vi "Strain with Nulling.vi"() -> ()   [LabVIEW 2009]
doc: "I. Description:\nThis example demonstrates how to acquire a continuous amount of data (Waveform) using the DAQ device's internal clock.\n\nII. Instructions for Running:\n1. Create an analog input voltage channel.\n2. Set the rate for the sample clock. Additionally, define the sample mode to be continuous.\n3. Call the Start VI to start the acquisition.\n4. Read the waveform data in a loop until the user hits the stop button or an error occurs.\nNote: This example reads data from one or more channels and returns an array of data. Use the Index Array function to access an individual channel of data.\n5. Call the Clear Task VI to clear the Task.\n6. Use the popup dialog box to display an error if any.\n\nIV. I/O Connections Overview:\nMake sure your signal input terminal matches the Physical Channel I/O Control. For further connection information, refer to your hardware reference manual."
uses:
  <vilib>/DAQmx/configure/timing.llb/DAQmx Timing (Sample Clock).vi
  <vilib>/DAQmx/create/channels.llb/DAQmx Create Channel (AI-Strain-Strain Gage).vi
  <vilib>/DAQmx/read.llb/DAQmx Read (Analog Wfm 1Chan NSamp).vi
  Program Files/National Instruments/LabVIEW 2009/resource/objmgr/daqmx.rc
panel:
  out "Strain Measurement":waveform(dbl)(graph)
  in  "Do Offset Nulling?":bool
  in  "Sample Rate":dbl=9.0 format="%0.2f"
  in  "strain gage information":T1={"gage factor"=2.0, "nominal gage resistance"=120.0, "poisson ratio"=0.3} {"poisson ratio" format="%0.2f"; "nominal gage resistance" format="%0.2f"; "gage factor" format="%0.2f"}
  in  "bridge information":T2={"strain configuration"=10271, "lead wire resistance"=0.0, "initial bridge voltage"=0.0, "voltage excitation source"=10200, "voltage excitation value"=2.5} {"initial bridge voltage" format="%0.2f"; "voltage excitation source" items=["Internal"=10200, "External"=10167, "None"=10230]; "voltage excitation value" format="%0.2f"; "lead wire resistance" format="%0.2f"; "strain configuration" items=["Full Bridge I"=10183, "Full Bridge II"=10184, "Full Bridge III"=10185, "Half Bridge I"=10188, "Half Bridge II"=10189, "Quarter Bridge I"=10271, "Quarter Bridge II"=10272]}
  in  "Strain Gage Channel":tag="cDAQ1Mod1/ai3" caption="Physical Channels"
  in  "minimum value (Strain)":dbl=-0.01 caption="Minimum Value" format="%0.3f"
  in  "maximum value (Strain)":dbl=0.01 caption="Maximum Value" format="%0.3f"
  in  "Samples to Read":i32=9
  in  "stop":bool
  # "Channel Parameters"
  # "Timing Parameters"
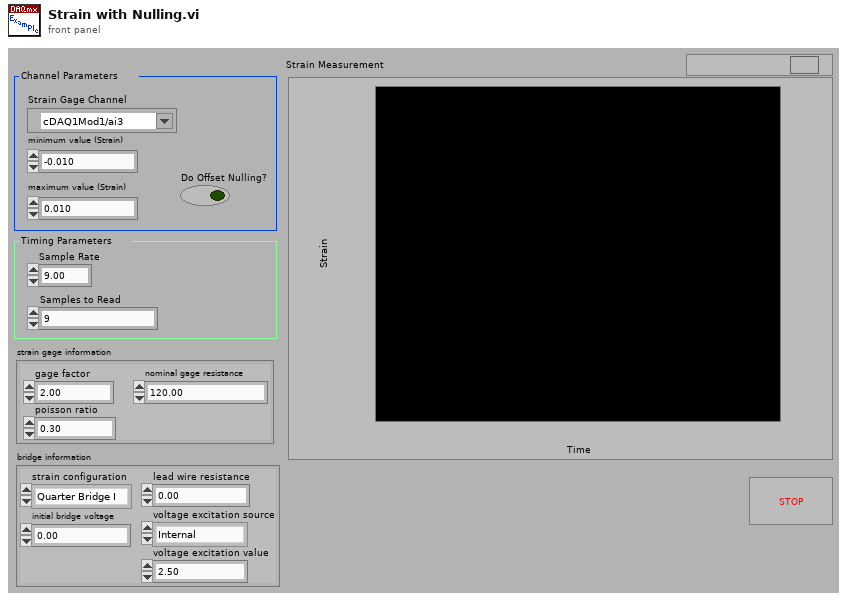
[diagram p1: front panel]
types:
  T1 = cluster{"gage factor":dbl, "nominal gage resistance":dbl, "poisson ratio":dbl}
  T2 = cluster{"strain configuration":i32, "lead wire resistance":dbl, "initial bridge voltage":dbl, "voltage excitation source":i32, "voltage excitation value":dbl}
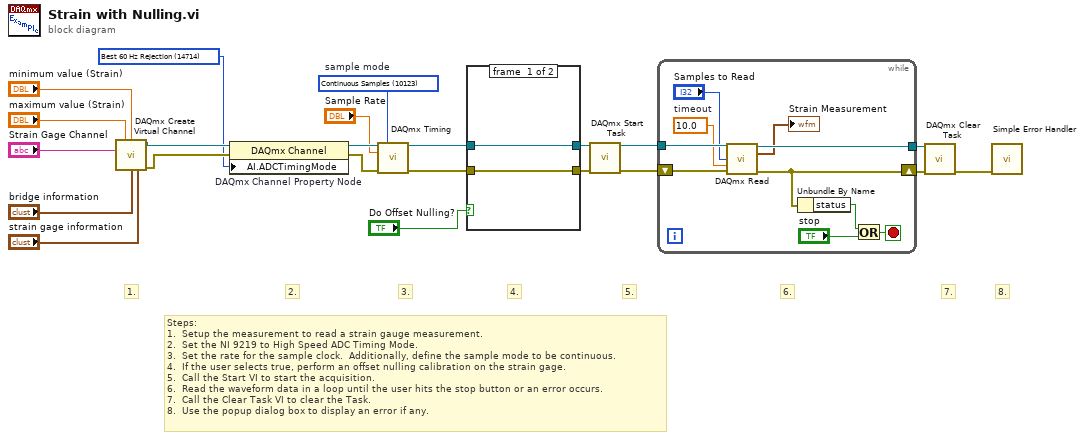
[diagram p0: block diagram]
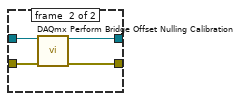
[diagram p2: hidden frame]
diagram:
  w9 = 14714 items=["High Resolution"=10195, "High Speed"=14712, "Best 50 Hz Rejection"=14713, "Best 60 Hz Rejection"=14714] ("AI.ADCTimingMode")
  w18 = 10123 items=["Finite Samples"=10178, "Continuous Samples"=10123]  # sample mode
  # "Steps: \n1.  Setup the measurement to read a strain gauge measurement.\n2.  Set the NI 9219 to High Speed ADC Timing Mode.\n3.  Set the rate for the sample clock.  Additionally, define the sample mode to be continuous.\n4.  If the user selects true, perform an offset nulling calibration on the strain gage.\n5.  Call the Start VI to start the acquisition.\n6.  Read the waveform data in a loop until the user hits the stop button or an error occurs.\n7.  Call the Clear Task VI to clear the Task.\n8.  Use the popup dialog box to display an error if any."
  # "4."
  # "6."
  # "2."
  # "8."
  # "7."
  # "5."
  # "3."
  # "1."
  n1 = call-poly <vilib>:"DAQmx Create Virtual Channel.vi"("maximum value"="maximum value (Strain)", "minimum value"="minimum value (Strain)", "physical channels"="Strain Gage Channel", "bridge information"="bridge information", "strain gage information"="strain gage information") -> ("task out"=w11:refnum<k21>, "error out"=w10:errorcluster)  [unwired: 9 in]
  n2 = property on="DAQmx Channel Property Node" class="DAQmx Channel"(reference=w11, error in=w10, "AI.ADCTimingMode"=w9) -> (reference out=w16:refnum<k21>, error out=w15:errorcluster)
  n3 = call-poly <vilib>:"DAQmx Timing.vi"("task/channels in"=w16, "sample mode"=w18, "rate"="Sample Rate", "error in"=w15) -> ("task out"=w4:refnum<k21>, "error out"=w2:errorcluster)  [unwired: 10 in]
  n4 = case shown="True" "Do Offset Nulling?" {
    tunnel: w4 -> [w24 w28]
    tunnel: [w24 w27] -> w3
    tunnel: w2 -> [w23 w26]
    tunnel: [w23 w25] -> w1
    frame #0 {
    }
    frame #1 {
      n5 = call <vilib>:"DAQmx Perform Bridge Offset Nulling Calibration.vi"("task/channels in"=w28, "error in"=w26) -> ("task out"=w27:refnum<k21>, "error out"=w25:errorcluster)  [unwired: 12 in]
    }
  }
  n6 = call <vilib>:"DAQmx Start Task.vi"("task/channels in"=w3, "error in"=w1) -> ("task out"=w20:refnum<k21>, "error out"=w22:errorcluster)  [unwired: 12 in]
  n7 = while {
    tunnel: w20 -> [w37]
    tunnel: [w36] -> w19
    shift-right: [w34] -> w17
    shift-left: w22 -> [w38]
    stop <- w32 stop-if-true
    w30 = 10.0  # timeout
    n8 = call-poly <vilib>:"DAQmx Read.vi"("task/channels in"=w37, "number of samples per channel"="Samples to Read", "timeout"=w30, "error in"=w38) -> ("task out"=w36:refnum<k21>, "data"=→"Strain Measurement":waveform(dbl), "error out"=w34:errorcluster)  [unwired: 9 in]
    n9 = Unbundle By Name "Unbundle By Name"(w34) -> ("status"=w33:bool)
    n10 = Or(x=w33, y="stop") -> (x .or. y?=w32:bool)
  }
  n11 = call <vilib>:"DAQmx Clear Task.vi"("task in"=w19, "error in"=w17) -> ("error out"=w21:errorcluster)  [unwired: 13 in]
  n12 = call <vilib>:"Simple Error Handler.vi"("error in (no error)"=w21) -> ()  [unwired: 4 in, 5 out]
